vi "Write MongoDB.Database.vi"(8 "error in (no error)":errorcluster, 10 "MongoDB.Database":refnum<k24>, 11 "MongoDB.Database in":refnum<class "MongoDB.Database.lvclass">) -> (0 "error out":errorcluster, 3 "MongoDB.Database out":refnum<class "MongoDB.Database.lvclass">)   [LabVIEW 2014, in "MongoDB.Database.lvclass"]
uses:
  MongoDB.Database.lvclass
  C:/Users/Richard/Documents/GitHub/mongo-labview-driver/CSharp/bin/MongoDB.Driver.Legacy.dll
  CSharp/bin/MongoDB.Driver.Legacy.dll
  MongoDB.Database.lvclass/MongoDB.Database.ctl
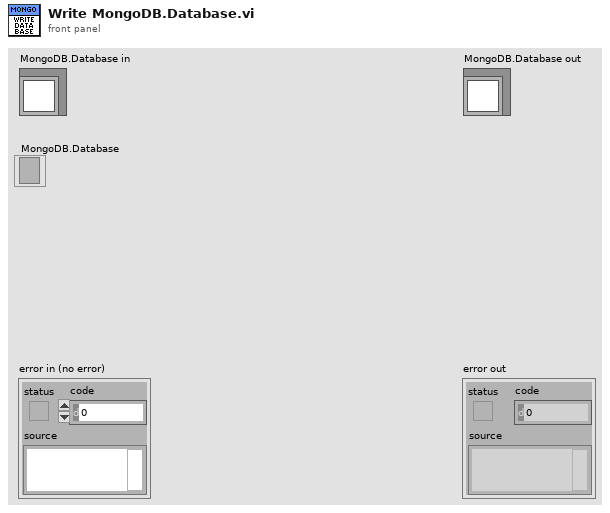
[diagram p1: front panel]
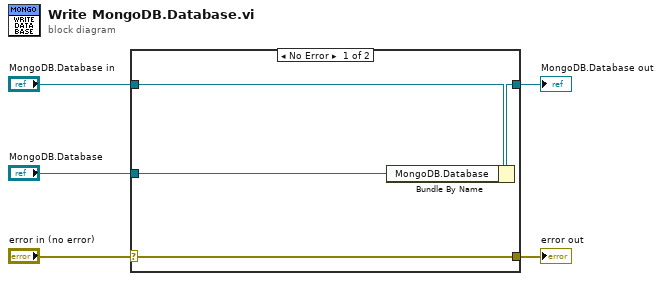
[diagram p0: block diagram]
diagram:
  n1 = case shown="No Error" "error in (no error)" {
    selector: "error in (no error)" -> [w9 w10]
    tunnel: [w9 w10] -> w4
    tunnel: [w7 w11] -> w2
    tunnel: "MongoDB.Database in" -> [w8 w11]
    tunnel: "MongoDB.Database" -> [w6 _]
    frame No Error {
      n2 = Bundle By Name(cluster=w8, "MongoDB.Database"=w6) -> (w7:refnum<class "MongoDB.Database.lvclass">)
    }
    frame Error {
    }
  }
  "error out" <- w4
  "MongoDB.Database out" <- w2
